vi "Begin.vi"(8 "error in":errorcluster) -> (0 "error out":errorcluster)   [LabVIEW 2020]
doc: "Called before other user functions, this VI is expected to open initial I/O refnums, load in file data, and do all program initialization. Notice that the <B>error out</B> terminal is simply used for data flow. Wiring it to other structures or subVIs ensures that this VI runs first."
uses:
  <vilib>/Rock Robotics/WPI/DriverStation/WPI_DriverStationRobotMode2.ctl
  <vilib>/Rock Robotics/WPI/Joystick/WPI_JoystickDeviceEnum.ctl
  <vilib>/Rock Robotics/WPI/RobotDrive/WPI_RobotDriveDevRef.ctl
  <vilib>/Rock Robotics/WPI/MotorControl/WPI_MotorControlDeviceRef.ctl
  <vilib>/Rock Robotics/WPI/MotorControl/WPI_MotorControlType.ctl
  <vilib>/Rock Robotics/SystemInterfaces/DIO/FPGA_DIOPWMChannel.ctl
  <vilib>/Rock Robotics/WPI/PWM/WPI_PWMDeadband.ctl
  <vilib>/Rock Robotics/SystemInterfaces/DIO/FPGA_DIOChannel.ctl
  <vilib>/Rock Robotics/WPI/SafetyOutput/WPI_SafetyOutputConfigMenu.ctl
  <vilib>/Rock Robotics/WPI/Compressor/WPI_CompressorFeedbackMode.ctl
  <vilib>/Rock Robotics/WPI/ThirdParty/REV Robotics/REVLib/Typedef/Spark MAX Control Type.ctl
  <vilib>/Rock Robotics/WPI/Solenoid/WPI_SolenoidChannel.ctl
  <vilib>/Rock Robotics/WPI/ThirdParty/REV Robotics/REVLib/Typedef/Spark MAX Motor Type.ctl
  <vilib>/Rock Robotics/WPI/ThirdParty/REV Robotics/REVLib/Typedef/Spark MAX Sensor Type.ctl
  Robot Global Data.vi
  <vilib>/Rock Robotics/Network Tables/NT Write String Array.vi
  <vilib>/Rock Robotics/WPI/RobotDrive/WPI_RobotDriveArcadeDrive_Standard(NoSaturation).vi
  <vilib>/Rock Robotics/WPI/Utilities/WPI_GetSetVariantRefNum.vi
  <vilib>/Rock Robotics/WPI/Solenoid/WPI_SolenoidOpenDouble.vi
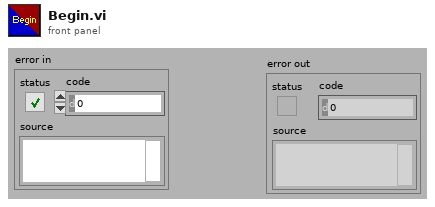
[diagram p1: front panel]
types:
  T1 = typedef "Spark MAX Sensor Type.ctl" = enum16{"No Sensor", "Hall Sensor", "Encoder", "-Not Available-", "Analog", "Alternate Encoder", "Duty Cycle"}
  T2 = cluster{"P Gain":dbl, "I Gain":dbl, "D Gain":dbl, "F Gain":dbl, "I Zone":dbl, "Min Output":dbl, "Max Output":dbl}
  T3 = typedef "FPGA_DIOChannel.ctl" = enum8{"DIO 0", "DIO 1", "DIO 2", "DIO 3", "DIO 4", "DIO 5", "DIO 6", "DIO 7", "DIO 8", "DIO 9", "DIO MXP 0", "DIO MXP 1", "DIO MXP 2", "DIO MXP 3", "DIO MXP 4", "DIO MXP 5", "DIO MXP 6", "DIO MXP 7", "DIO MXP 8", "DIO MXP 9", "DIO MXP 10", "DIO MXP 11", "DIO MXP 12", "DIO MXP 13", "DIO MXP 14", "DIO MXP 15", "SPI Port CS1", "SPI Port CS2", "SPI Port CS3", "SPI Port MISO", "SPI Port MOSI", "Invalid"}
  T4 = typedef "WPI_SolenoidChannel.ctl" = enum8{"Solenoid 0", "Solenoid 1", "Solenoid 2", "Solenoid 3", "Solenoid 4", "Solenoid 5", "Solenoid 6", "Solenoid 7", "Solenoid 8", "Solenoid 9", "Solenoid 10", "Solenoid 11", "Solenoid 12", "Solenoid 13", "Solenoid 14", "Solenoid 15", "Invalid"}
  T5 = typedef "Spark MAX Control Type.ctl" = enum16{"Percent VBus", "Voltage", "Velocity", "Position", "Smart Motion", "Current", "Smart Velocity"}
  T6 = typedef "Spark MAX Motor Type.ctl" = enum16{"Brushed", "Brushless"}
  T7 = typedef "WPI_CompressorFeedbackMode.ctl" = enum16{"Analog Only", "Digital Only", "Hybrid"}
  T8 = cluster{"Feedback Sensor":T7, "Max Pressure (PSI)":dbl, "Min Pressure (PSI)":dbl}
  T9 = typedef "WPI_JoystickDeviceEnum.ctl" = enum16{"USB 0", "USB 1", "USB 2", "USB 3", "USB 4", "USB 5"}
  T10 = typedef "FPGA_DIOPWMChannel.ctl" = enum8{"PWM 0", "PWM 1", "PWM 2", "PWM 3", "PWM 4", "PWM 5", "PWM 6", "PWM 7", "PWM 8", "PWM 9", "PWM MXP 0", "PWM MXP 1", "PWM MXP 2", "PWM MXP 3", "PWM MXP 4", "PWM MXP 5", "PWM MXP 6", "PWM MXP 7", "PWM MXP 8", "PWM MXP 9", "Invalid"}
  T11 = typedef "WPI_SafetyOutputConfigMenu.ctl" = enum16{"Enable", "Disable"}
  T12 = typedef "WPI_RobotDriveDevRef.ctl" = cluster{"DevStatus":errorcluster, "Motors[]":T13[], "Square Inputs":bool, "Max Output":dbl}
  T13 = typedef "WPI_MotorControlDeviceRef.ctl" = cluster{"DeviceStatus":errorcluster, "Type":T14, "PWM":cluster{"PWM Channel":T10, "DeadBand":T15}, "CAN":cluster{"Device Number":u8, "SetOutput VI Ref":variant, "GetOutput VI Ref":variant, "Enable VI Ref":variant, "Disable VI Ref":variant, "Data":variant}, "Invert":bool, "DIO PWM":cluster{"PWM \"Enable\" Channel":T10, "DIOChannel":T3, "PWM Rate":dbl}}
  T14 = typedef "WPI_MotorControlType.ctl" = enum16{"PWM", "CAN", "DIO PWM"}
  T15 = typedef "WPI_PWMDeadband.ctl" = cluster{"Name":string, "maxPositivePwm":i32, "minPositivePwm":i32, "centerPwm":i32, "maxNegativePwm":i32, "minNegativePwm":i32, "angularRange":u16}
  T16 = typedef "WPI_DriverStationRobotMode2.ctl" = enum16{"Autonomous Disabled", "Autonomous Enabled", "Teleop Disabled", "Teleop Enabled", "Disconnected", "Finish", "Test Disabled", "Test Enabled", "Emergency Stopped"}
  T17 = typedef "WPI_PWMDeviceRef.ctl" = cluster{"DeviceStatus":errorcluster, "PWM Channel":T10}
  T18 = typedef "WPI_SolenoidDevRef.ctl" = cluster{"DevStatus":errorcluster, "Pneumatics Control Module":u8, "Forward Solenoid Channel":T4, "Reverse Solenoid Channel":T4}
  T19 = typedef "CTRE_PigeonIMU_DeviceRef.ctl" = cluster{"DeviceStatus":errorcluster, "Device Number":u8, "Type":T20, "Device ID":u32, "Handle":u64, "UsageFrame":u32, "Library Path":path}
  T20 = typedef "CTRE_PigeonIMU_ConnectionType.ctl" = u32
  T21 = typedef "WPI_JoystickDevRef.ctl" = cluster{"Device":T9}
  T22 = typedef "WPI_CompressorDevRef.ctl" = cluster{"DevStatus":errorcluster, "Pneumatics Control Module":u8}
  T23 = typedef "WPI_DigitalInputDevRef.ctl" = cluster{"DevStatus":errorcluster, "DIO Channel":T3}
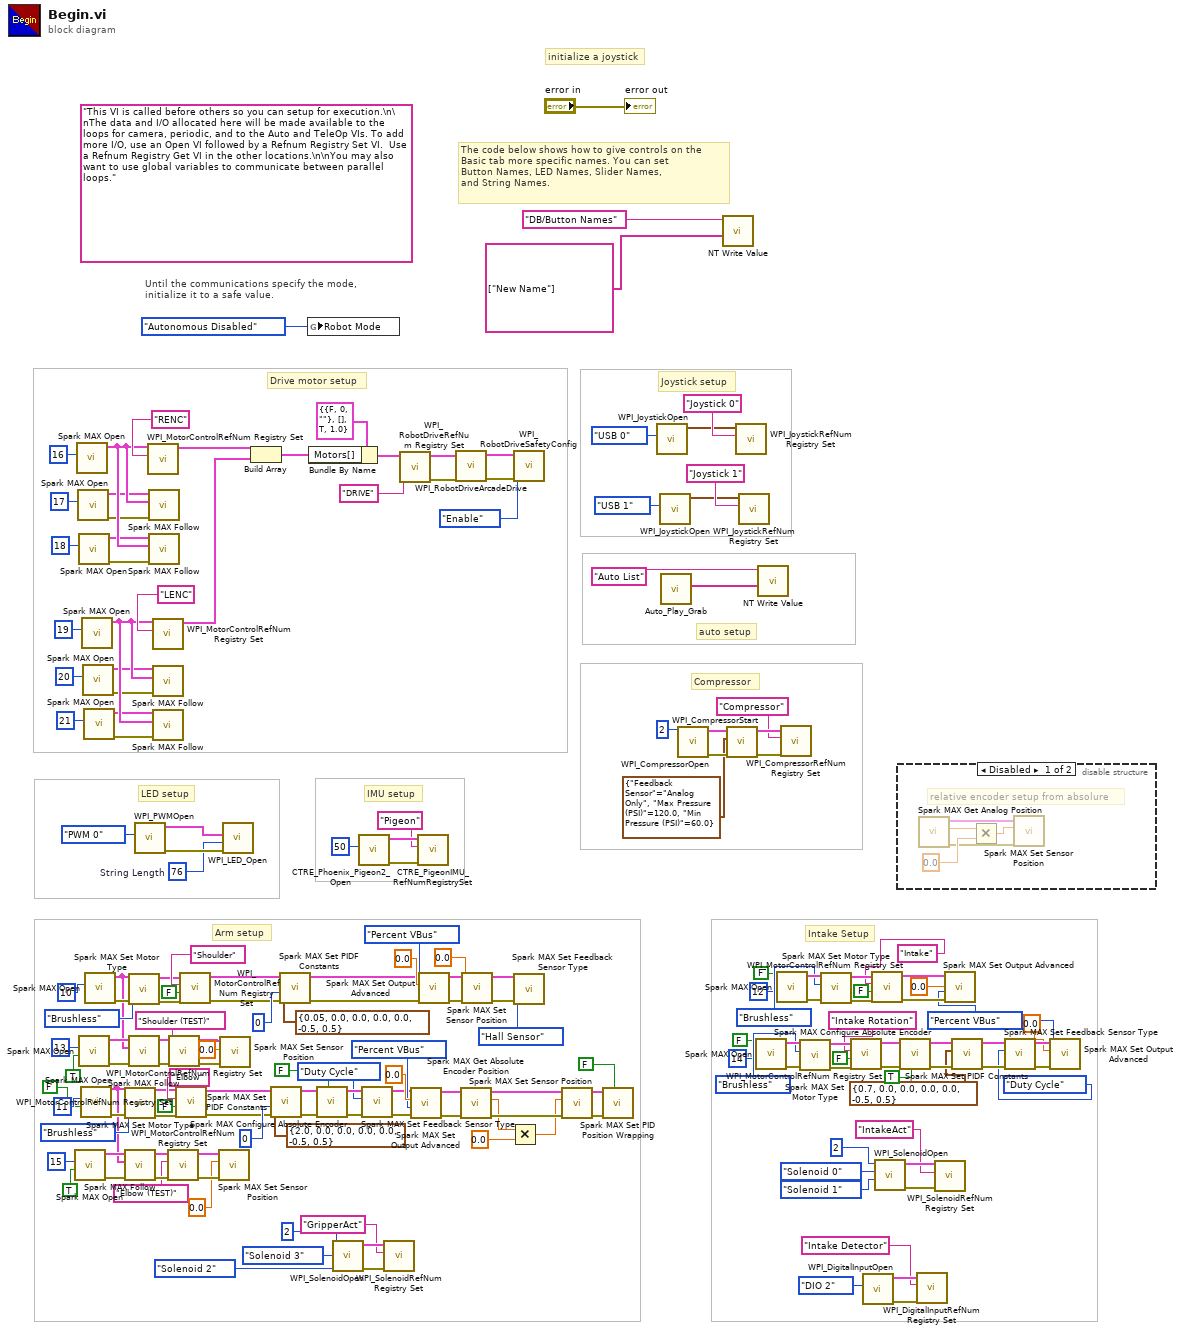
[diagram p0: block diagram]
diagram:
  w35 = Spark_MAX_Control_Type."Percent VBus" ("Control Mode")
  w156 = u16 76  # String Length
  (unwired) "This VI is called before others so you can setup for execution.\n\nThe data and I/O allocated here will be made available to the loops for camera, periodic, and to the Auto and TeleOp VIs. To add more I/O, use an Open VI followed by a Refnum Registry Set VI.  Use a Refnum Registry Get VI in the other locations.\n\nYou may also want to use global variables to communicate between parallel loops."
  # "Intake Setup"
  # "Arm setup"
  # "Compressor"
  # "IMU setup"
  # "auto setup"
  # "Joystick setup"
  # "LED setup"
  # "Drive motor setup"
  # "The code below shows how to give controls on the\nBasic tab more specific names. You can set\nButton Names, LED Names, Slider Names,\nand String Names."
  # "initialize a joystick"
  # "Until the communications specify the mode,\ninitialize it to a safe value."
  n1 = call <vilib>:"Spark MAX Open.vi"("Invert"=TRUE, "Device Number"=u8 15) -> ("error out"=w101:errorcluster, "MotorControlDeviceRef"=w102:T13)  [unwired: 8 in]
  n2 = call <vilib>:"Spark MAX Open.vi"("Device Number"=u8 16) -> ("MotorControlDeviceRef"=w146:T13)  [unwired: 9 in, 1 out]
  n3 = call <vilib>:"Spark MAX Open.vi"("Device Number"=u8 17) -> ("error out"=w141:errorcluster, "MotorControlDeviceRef"=w142:T13)  [unwired: 9 in]
  n4 = call <vilib>:"Spark MAX Open.vi"("Device Number"=u8 18) -> ("error out"=w140:errorcluster, "MotorControlDeviceRef"=w139:T13)  [unwired: 9 in]
  n5 = call <vilib>:"Spark MAX Open.vi"("Invert"=TRUE, "Device Number"=u8 13) -> ("error out"=w105:errorcluster, "MotorControlDeviceRef"=w106:T13)  [unwired: 8 in]
  n6 = call <vilib>:"Spark MAX Open.vi"("Invert"=FALSE, "Device Number"=u8 11) -> ("error out"=w116:errorcluster, "MotorControlDeviceRef"=w100:T13)  [unwired: 8 in]
  n7 = call <vilib>:"Spark MAX Open.vi"("Device Number"=u8 19) -> ("MotorControlDeviceRef"=w145:T13)  [unwired: 9 in, 1 out]
  n8 = call <vilib>:"Spark MAX Open.vi"("Device Number"=u8 20) -> ("error out"=w135:errorcluster, "MotorControlDeviceRef"=w136:T13)  [unwired: 9 in]
  n9 = call <vilib>:"Spark MAX Open.vi"("Device Number"=u8 21) -> ("error out"=w133:errorcluster, "MotorControlDeviceRef"=w134:T13)  [unwired: 9 in]
  n10 = call <vilib>:"Spark MAX Open.vi"("Device Number"=u8 10) -> ("error out"=w123:errorcluster, "MotorControlDeviceRef"=w104:T13)  [unwired: 9 in]
  n11 = call <vilib>:"Spark MAX Set Motor Type.vi"("error in (no error)"=w116, "Motor Type"=Spark_MAX_Motor_Type."Brushless", "MotorControlDevRef"=w100) -> ("error out"=w114:errorcluster, "MotorControlDeviceRef"=w115:T13)  [unwired: 7 in]
  n12 = call <vilib>:"Spark MAX Follow.vi"("error in (no error)"=w101, "Master Controller"=w100, "MotorControlDeviceRef"=w102) -> ("error out"=w94:errorcluster, "MotorControlDeviceRef"=w95:T13)  [unwired: 7 in]
  n13 = call <vilib>:"Spark MAX Set Motor Type.vi"("error in (no error)"=w123, "Motor Type"=Spark_MAX_Motor_Type."Brushless", "MotorControlDevRef"=w104) -> ("error out"=w121:errorcluster, "MotorControlDeviceRef"=w122:T13)  [unwired: 7 in]
  n14 = call <vilib>:"Spark MAX Follow.vi"("error in (no error)"=w105, "Master Controller"=w104, "MotorControlDeviceRef"=w106) -> ("error out"=w91:errorcluster, "MotorControlDeviceRef"=w92:T13)  [unwired: 7 in]
  n15 = call <vilib>:"WPI_PWMOpen.vi"("PWM Channel"=FPGA_DIOPWMChannel."PWM 0") -> ("error out"=w157:errorcluster, "PWMDeviceRef"=w158:T17)  [unwired: 9 in]
  n16 = call <vilib>:"WPI_MotorControlRefNum Registry Set.vi"("refnum name"="RENC", "MotorControlDevRef"=w146) -> ("MotorControlDevRef"=w168:T13)  [unwired: 8 in, 1 out]
  n17 = call <vilib>:"Spark MAX Follow.vi"("error in (no error)"=w141, "Master Controller"=w146, "MotorControlDeviceRef"=w142) -> ()  [unwired: 7 in, 2 out]
  n18 = call <vilib>:"Spark MAX Follow.vi"("error in (no error)"=w140, "Master Controller"=w146, "MotorControlDeviceRef"=w139) -> ()  [unwired: 7 in, 2 out]
  n19 = call <vilib>:"WPI_MotorControlRefNum Registry Set.vi"("refnum name"="LENC", "MotorControlDevRef"=w145) -> ("MotorControlDevRef"=w167:T13)  [unwired: 8 in, 1 out]
  n20 = call <vilib>:"Spark MAX Follow.vi"("error in (no error)"=w135, "Master Controller"=w145, "MotorControlDeviceRef"=w136) -> ()  [unwired: 7 in, 2 out]
  n21 = call <vilib>:"Spark MAX Follow.vi"("error in (no error)"=w133, "Master Controller"=w145, "MotorControlDeviceRef"=w134) -> ()  [unwired: 7 in, 2 out]
  n22 = call <vilib>:"WPI_MotorControlRefNum Registry Set.vi"("error in (no error)"=w94, "refnum name"="Elbow (TEST)", "MotorControlDevRef"=w95) -> ("error out"=w81:errorcluster, "MotorControlDevRef"=w82:T13)  [unwired: 7 in]
  n23 = call <vilib>:"WPI_MotorControlRefNum Registry Set.vi"("error in (no error)"=w91, "refnum name"="Shoulder (TEST)", "MotorControlDevRef"=w92) -> ("error out"=w78:errorcluster, "MotorControlDevRef"=w79:T13)  [unwired: 7 in]
  n24 = call <vilib>:"WPI_MotorControlRefNum Registry Set.vi"("error in (no error)"=w114, "Test Mode Only"=FALSE, "refnum name"="Elbow", "MotorControlDevRef"=w115) -> ("error out"=w65:errorcluster, "MotorControlDevRef"=w66:T13)  [unwired: 6 in]
  n25 = call <vilib>:"WPI_MotorControlRefNum Registry Set.vi"("error in (no error)"=w121, "Test Mode Only"=FALSE, "refnum name"="Shoulder", "MotorControlDevRef"=w122) -> ("error out"=w67:errorcluster, "MotorControlDevRef"=w68:T13)  [unwired: 6 in]
  n26 = call <vilib>:"Spark MAX Set Sensor Position.vi"("error in"=w81, "Position"=0.0, "MotorControlDeviceRef"=w82) -> ()  [unwired: 7 in, 2 out]
  n27 = call <vilib>:"Spark MAX Set Sensor Position.vi"("error in"=w78, "Position"=0.0, "MotorControlDeviceRef"=w79) -> ()  [unwired: 7 in, 2 out]
  n28 = call <vilib>:"WPI_LED_Open.vi"("error in"=w157, "String Length"=w156, "PWMDeviceRef"=w158) -> ()  [unwired: 8 in, 1 out]
  n29 = Build Array(w168, w167) -> (w166:T13[])
  n30 = call <vilib>:"Spark MAX Set PIDF Constants.vi"("error in"=w65, "PIDF Slot"=0, "PID Constants"=T2 {"P Gain"=2.0, "I Gain"=0.0, "D Gain"=0.0, "F Gain"=0.0, "I Zone"=0.0, "Min Output"=-0.5, "Max Output"=0.5}, "MotorControlDeviceRef"=w66) -> ("error out"=w74:errorcluster, "MotorControlDeviceRef"=w75:T13)  [unwired: 6 in]
  n31 = call <vilib>:"Spark MAX Set PIDF Constants.vi"("error in"=w67, "PIDF Slot"=0, "PID Constants"=T2 {"P Gain"=0.05, "I Gain"=0.0, "D Gain"=0.0, "F Gain"=0.0, "I Zone"=0.0, "Min Output"=-0.5, "Max Output"=0.5}, "MotorControlDeviceRef"=w68) -> ("error out"=w9:errorcluster, "MotorControlDeviceRef"=w10:T13)  [unwired: 6 in]
  n32 = global write "Robot Global Data.vi" "Robot Mode"(WPI_DriverStationRobotMode2."Autonomous Disabled" ("Robot Mode")) -> ()
  n33 = Bundle By Name(cluster=T12 {"DevStatus"={"status"=FALSE, "code"=0, "source"=""}, "Motors[]"=[], "Square Inputs"=TRUE, "Max Output"=1.0} ("RobotDriveDevRef"), "Motors[]"=w166) -> (w165:T12)
  n34 = call <vilib>:"Spark MAX Configure Absolute Encoder.vi"("Inverted (F)"=FALSE, "error in (no error)"=w74, "MotorControlDeviceRef in"=w75) -> ("error out"=w72:errorcluster, "MotorControlDeviceRef out"=w73:T13)  [unwired: 7 in]
  n35 = call-poly <vilib>:"WPI_SolenoidOpen.vi"("Reverse Solenoid Channel"=WPI_SolenoidChannel."Solenoid 2", "Forward Solenoid Channel"=WPI_SolenoidChannel."Solenoid 3" ("Solenoid Channel"), "Pneumatics Device (def)"=u8 2) -> ("error out"=w88:errorcluster, "SolenoidDevRef"=w87:T18)  [unwired: 7 in]
  n36 = call <vilib>:"CTRE_Phoenix_Pigeon2_Open.vi"("Device Number"=u8 50) -> ("error out"=w150:errorcluster, "PigeonIMUDevRef"=w149:T19)  [unwired: 9 in]
  n37 = call <vilib>:"Spark MAX Set Feedback Sensor Type.vi"("error in (no error)"=w72, "Sensor Type"=Spark_MAX_Sensor_Type."Duty Cycle", "MotorControlDevRef"=w73) -> ("error out"=w69:errorcluster, "MotorControlDeviceRef"=w70:T13)  [unwired: 7 in]
  n38 = call <vilib>:"WPI_SolenoidRefNum Registry Set.vi"("error in (no error)"=w88, "refnum name"="GripperAct", "SolenoidDevRef"=w87) -> ()  [unwired: 7 in, 2 out]
  n39 = call <vilib>:"WPI_RobotDriveRefNum Registry Set.vi"("refnum name"="DRIVE", "RobotDriveDevRef"=w165) -> ("error out"=w162:errorcluster, "RobotDriveDevRef"=w163:T12)  [unwired: 8 in]
  n40 = call <vilib>:"Spark MAX Set Output Advanced.vi"("error in (no error)"=w69, "Control Mode"=Spark_MAX_Control_Type."Percent VBus", "Setpoint"=0.0, "MotorControlDevRef"=w70) -> ("error out"=w63:errorcluster, "MotorControlDevRef"=w64:T13)  [unwired: 6 in]
  n41 = call <vilib>:"CTRE_PigeonIMU_RefNumRegistrySet.vi"("error in (no error)"=w150, "refnum name"="Pigeon", "PigeonIMUDevRef"=w149) -> ()  [unwired: 7 in, 2 out]
  n42 = call <vilib>:"Spark MAX Set Output Advanced.vi"("error in (no error)"=w9, "Control Mode"=Spark_MAX_Control_Type."Percent VBus", "Setpoint"=0.0, "MotorControlDevRef"=w10) -> ("error out"=w11:errorcluster, "MotorControlDevRef"=w12:T13)  [unwired: 6 in]
  n43 = call-poly <vilib>:"WPI_RobotDriveArcadeDrive.vi"("error in (no error)"=w162, "RobotDriveDevRef"=w163) -> ("error out"=w161:errorcluster, "RobotDriveDevRef"=w160:T12)  [unwired: 7 in, 1 out]
  n44 = call <vilib>:"Spark MAX Get Absolute Encoder Position.vi"("error in (no error)"=w63, "MotorControlDeviceRef in"=w64) -> ("error out"=w61:errorcluster, "Position"=w60:dbl, "MotorControlDeviceRef out"=w62:T13)  [unwired: 6 in, 1 out]
  n45 = call <vilib>:"Spark MAX Set Sensor Position.vi"("error in"=w11, "Position"=0.0, "MotorControlDeviceRef"=w12) -> ("error out"=w6:errorcluster, "MotorControlDeviceRef"=w7:T13)  [unwired: 7 in]
  n46 = Multiply(x=w60, y=0.0) -> (x*y=w59:dbl)
  n47 = call <vilib>:"WPI_RobotDriveSafetyConfig.vi"("error in (no error)"=w161, "mode"=WPI_SafetyOutputConfigMenu."Enable", "RobotDriveDevRef"=w160) -> ()  [unwired: 7 in, 2 out]
  n48 = call <vilib>:"Spark MAX Set Feedback Sensor Type.vi"("error in (no error)"=w6, "Sensor Type"=Spark_MAX_Sensor_Type."Hall Sensor", "MotorControlDevRef"=w7) -> ()  [unwired: 7 in, 2 out]
  n49 = call <vilib>:"Spark MAX Set Sensor Position.vi"("error in"=w61, "Position"=w59, "MotorControlDeviceRef"=w62) -> ("error out"=w4:errorcluster, "MotorControlDeviceRef"=w3:T13)  [unwired: 7 in]
  n50 = call <vilib>:"Spark MAX Set PID Position Wrapping.vi"("Enable (F)"=FALSE, "error in (no error)"=w4, "MotorControlDeviceRef in"=w3) -> ()  [unwired: 7 in, 2 out]
  n51 = call <vilib>:"WPI_JoystickOpen.vi"("JoystickDevice"=WPI_JoystickDeviceEnum."USB 0") -> ("JoystickDevRef"=w179:T21)  [unwired: 10 in]
  n52 = call <vilib>:"WPI_JoystickOpen.vi"("JoystickDevice"=WPI_JoystickDeviceEnum."USB 1") -> ("JoystickDevRef"=w153:T21)  [unwired: 10 in]
  n53 = call "Auto_Play_Grab.vi"() -> ("Auto Plays"=w151:string[])  [unwired: 10 in, 1 out]
  n54 = call <vilib>:"WPI_CompressorOpen.vi"("Pneumatics device (def)"=u8 2) -> ("CompressorDevRef"=w131:T22, "error out"=w132:errorcluster)  [unwired: 13 in]
  n55 = call-poly <vilib>:"NT Write Value.vi"("value"=string[] ["New Name"], "name"="DB/Button Names" ("Name")) -> ()  [unwired: 9 in, 1 out]
  n56 = call <vilib>:"WPI_CompressorStart.vi"("error in (no error)"=w132, "Feedback Configuration"=T8 {"Feedback Sensor"=enum."Analog Only", "Max Pressure (PSI)"=120.0, "Min Pressure (PSI)"=60.0}, "CompressorDevRef"=w131) -> ("error out"=w129:errorcluster, "CompressorDevRef"=w128:T22)  [unwired: 7 in]
  n57 = call <vilib>:"WPI_JoystickRefNum Registry Set.vi"("refnum name"="Joystick 0", "JoystickDevRef"=w179) -> ()  [unwired: 8 in, 2 out]
  n58 = call <vilib>:"WPI_JoystickRefNum Registry Set.vi"("refnum name"="Joystick 1", "JoystickDevRef"=w153) -> ()  [unwired: 8 in, 2 out]
  n59 = call <vilib>:"Spark MAX Open.vi"("Invert"=FALSE, "Device Number"=u8 14) -> ("error out"=w40:errorcluster, "MotorControlDeviceRef"=w43:T13)  [unwired: 8 in]
  n60 = call-poly <vilib>:"NT Write Value.vi"("value"=w151, "name"="Auto List" ("Name")) -> ()  [unwired: 9 in, 1 out]
  n61 = call <vilib>:"Spark MAX Open.vi"("Invert"=FALSE, "Device Number"=u8 12) -> ("error out"=w36:errorcluster, "MotorControlDeviceRef"=w39:T13)  [unwired: 8 in]
  n62 = call <vilib>:"WPI_CompressorRefNum Registry Set.vi"("error in (no error)"=w129, "refnum name"="Compressor", "CompressorDevRef"=w128) -> ()  [unwired: 7 in, 2 out]
  n63 = call <vilib>:"Spark MAX Set Motor Type.vi"("error in (no error)"=w40, "Motor Type"=Spark_MAX_Motor_Type."Brushless", "MotorControlDevRef"=w43) -> ("error out"=w42:errorcluster, "MotorControlDeviceRef"=w41:T13)  [unwired: 7 in]
  n64 = call <vilib>:"Spark MAX Set Motor Type.vi"("error in (no error)"=w36, "Motor Type"=Spark_MAX_Motor_Type."Brushless", "MotorControlDevRef"=w39) -> ("error out"=w38:errorcluster, "MotorControlDeviceRef"=w37:T13)  [unwired: 7 in]
  n65 = call <vilib>:"WPI_MotorControlRefNum Registry Set.vi"("error in (no error)"=w42, "Test Mode Only"=FALSE, "refnum name"="Intake Rotation", "MotorControlDevRef"=w41) -> ("error out"=w55:errorcluster, "MotorControlDevRef"=w54:T13)  [unwired: 6 in]
  n66 = call <vilib>:"WPI_DigitalInputOpen.vi"("DIO Channel"=FPGA_DIOChannel."DIO 2") -> ("error out"=w48:errorcluster, "DigitalInputDevRef"=w49:T23)  [unwired: 9 in]
  n67 = call <vilib>:"WPI_MotorControlRefNum Registry Set.vi"("error in (no error)"=w38, "Test Mode Only"=FALSE, "refnum name"="Intake", "MotorControlDevRef"=w37) -> ("error out"=w44:errorcluster, "MotorControlDevRef"=w45:T13)  [unwired: 6 in]
  n68 = call-poly <vilib>:"WPI_SolenoidOpen.vi"("Reverse Solenoid Channel"=WPI_SolenoidChannel."Solenoid 1", "Forward Solenoid Channel"=WPI_SolenoidChannel."Solenoid 0", "Pneumatics Device (def)"=u8 2) -> ("error out"=w46:errorcluster, "SolenoidDevRef"=w47:T18)  [unwired: 7 in]
  n69 = disable-structure shown="Disabled" {
    frame Disabled {
      # "relative encoder setup from absolure"
      n70 = call <vilib>:"Spark MAX Get Analog Position.vi"() -> ("error out"=w182:errorcluster, "Analog Position"=w186:dbl, "MotorControlDevRef out"=w183:T13)  [unwired: 8 in, 1 out]
      n71 = Multiply(x=w186, y=0.0) -> (x*y=w184:dbl)
      n72 = call <vilib>:"Spark MAX Set Sensor Position.vi"("error in"=w182, "Position"=w184, "MotorControlDeviceRef"=w183) -> ()  [unwired: 7 in, 2 out]
    }
    frame Enabled {
    }
  }
  n73 = call <vilib>:"Spark MAX Configure Absolute Encoder.vi"("Inverted (F)"=TRUE, "error in (no error)"=w55, "MotorControlDeviceRef in"=w54) -> ("error out"=w50:errorcluster, "MotorControlDeviceRef out"=w51:T13)  [unwired: 7 in]
  n74 = call <vilib>:"WPI_DigitalInputRefNum Registry Set.vi"("error in (no error)"=w48, "refnum name"="Intake Detector", "DigitalInputDevRef"=w49) -> ()  [unwired: 7 in, 2 out]
  n75 = call <vilib>:"WPI_SolenoidRefNum Registry Set.vi"("error in (no error)"=w46, "refnum name"="IntakeAct", "SolenoidDevRef"=w47) -> ()  [unwired: 7 in, 2 out]
  n76 = call <vilib>:"Spark MAX Set Output Advanced.vi"("error in (no error)"=w44, "Control Mode"=w35, "Setpoint"=0.0, "MotorControlDevRef"=w45) -> ()  [unwired: 6 in, 2 out]
  n77 = call <vilib>:"Spark MAX Set PIDF Constants.vi"("error in"=w50, "PID Constants"=T2 {"P Gain"=0.7, "I Gain"=0.0, "D Gain"=0.0, "F Gain"=0.0, "I Zone"=0.0, "Min Output"=-0.5, "Max Output"=0.5}, "MotorControlDeviceRef"=w51) -> ("error out"=w52:errorcluster, "MotorControlDeviceRef"=w53:T13)  [unwired: 7 in]
  n78 = call <vilib>:"Spark MAX Set Feedback Sensor Type.vi"("error in (no error)"=w52, "Sensor Type"=Spark_MAX_Sensor_Type."Duty Cycle", "MotorControlDevRef"=w53) -> ("error out"=w56:errorcluster, "MotorControlDeviceRef"=w57:T13)  [unwired: 7 in]
  n79 = call <vilib>:"Spark MAX Set Output Advanced.vi"("error in (no error)"=w56, "Control Mode"=w35, "Setpoint"=0.0, "MotorControlDevRef"=w57) -> ()  [unwired: 6 in, 2 out]
  "error out" <- "error in"
